vi "setTriggerControl.vi"(10 "TriggerControl":refnum<class "IBooleanControl.lvclass">, 11 "ILCCommunications in":refnum<class "ILCCommunications.lvclass">) -> (3 "ILCCommunications out":refnum<class "ILCCommunications.lvclass">)   [LabVIEW 2016]
uses:
  ILCCommunications.lvclass
  Common_RT_FPGA/IBooleanControl/IBooleanControl.lvclass
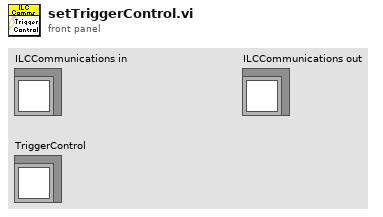
[diagram p1: front panel]
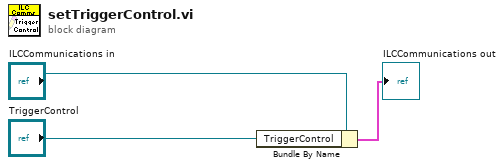
[diagram p0: block diagram]
diagram:
  n1 = Bundle By Name(cluster="ILCCommunications in", "TriggerControl"="TriggerControl") -> (→"ILCCommunications out":cluster{})
